vi "AddTestMethod_Item_Interface.vi"() -> (3 "InterfaceTable":T1)   [LabVIEW 2013]
uses:
  <resource>/Framework/Providers/API/Item_Interface.ctl
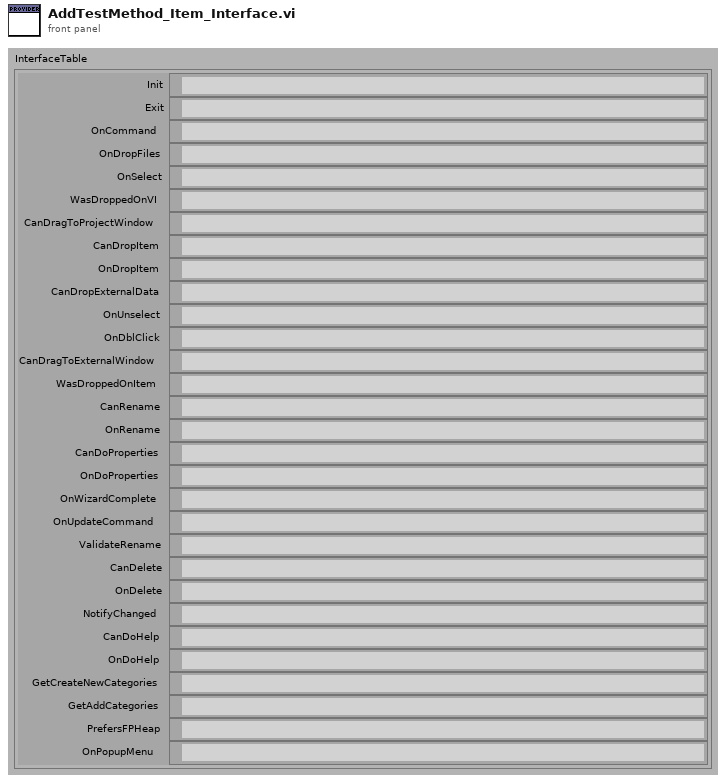
[diagram p1: front panel]
types:
  T1 = typedef "Item_Interface.ctl" = cluster{"Init":path, "Exit":path, "OnCommand":path, "OnDropFiles":path, "OnSelect":path, "WasDroppedOnVI":path, "CanDragToProjectWindow":path, "CanDropItem":path, "OnDropItem":path, "CanDropExternalData":path, "OnUnselect":path, "OnDblClick":path, "CanDragToExternalWindow":path, "WasDroppedOnItem":path, "CanRename":path, "OnRename":path, "CanDoProperties":path, "OnDoProperties":path, "OnWizardComplete":path, "OnUpdateCommand":path, "ValidateRename":path, "CanDelete":path, "OnDelete":path, "NotifyChanged":path, "CanDoHelp":path, "OnDoHelp":path, "GetCreateNewCategories":path, "GetAddCategories":path, "PrefersFPHeap":path, "OnPopupMenu":path}
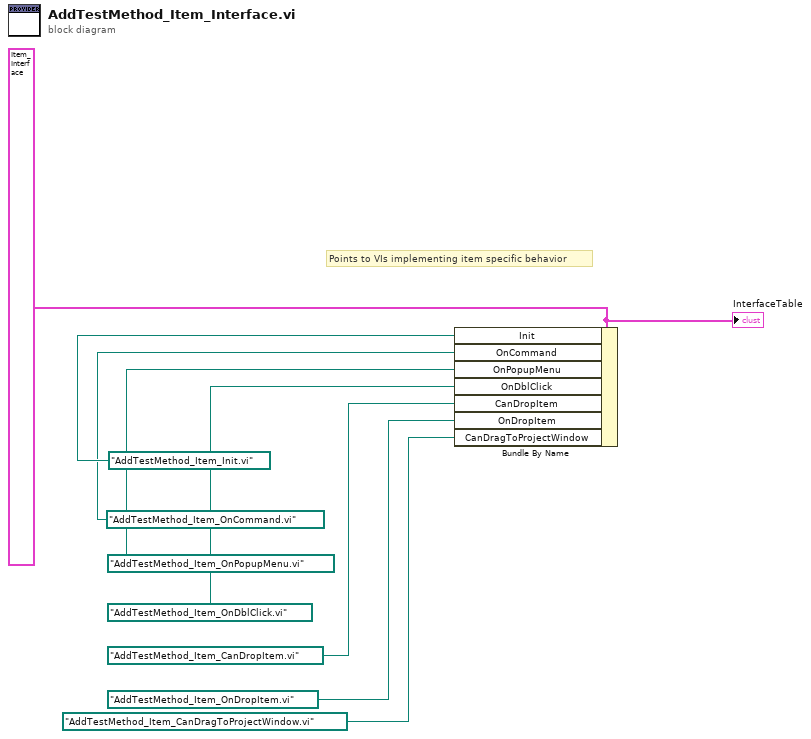
[diagram p0: block diagram]
diagram:
  w1 = T1 {"Init"=path "", "Exit"=path "", "OnCommand"=path "", "OnDropFiles"=path "", "OnSelect"=path "", "WasDroppedOnVI"=path "", "CanDragToProjectWindow"=path "", "CanDropItem"=path "", "OnDropItem"=path "", "CanDropExternalData"=path "", "OnUnselect"=path "", "OnDblClick"=path "", "CanDragToExternalWindow"=path "", "WasDroppedOnItem"=path "", "CanRename"=path "", "OnRename"=path "", "CanDoProperties"=path "", "OnDoProperties"=path "", "OnWizardComplete"=path "", "OnUpdateCommand"=path "", "ValidateRename"=path "", "CanDelete"=path "", "OnDelete"=path "", "NotifyChanged"=path "", "CanDoHelp"=path "", "OnDoHelp"=path "", "GetCreateNewCategories"=path "", "GetAddCategories"=path "", "PrefersFPHeap"=path "", "OnPopupMenu"=path ""} ("InterfaceTable")
  # "Points to VIs implementing item specific behavior"
  n1 = Bundle By Name(cluster=w1, "Init"=path "AddTestMethod_Item_Init.vi", "OnCommand"=path "AddTestMethod_Item_OnCommand.vi", "OnPopupMenu"=path "AddTestMethod_Item_OnPopupMenu.vi", "OnDblClick"=path "AddTestMethod_Item_OnDblClick.vi", "CanDropItem"=path "AddTestMethod_Item_CanDropItem.vi", "OnDropItem"=path "AddTestMethod_Item_OnDropItem.vi", "CanDragToProjectWindow"=path "AddTestMethod_Item_CanDragToProjectWindow.vi") -> ()  [unwired: 1 out]
  "InterfaceTable" <- w1
